vi "Open Reference (Simulate).vi"(8 "error in (no error)":errorcluster, 11 "Instrument Refnum in":refnum<visa-resource-name>) -> (0 "error out":errorcluster, 3 "Instrument Refnum out":refnum<visa-resource-name>)   [LabVIEW 2012]
doc: "Simulates initializing a hardware reference"
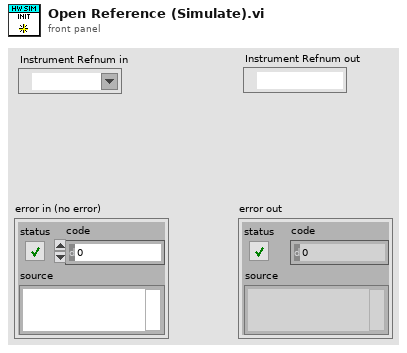
[diagram p1: front panel]
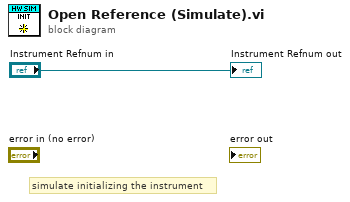
[diagram p0: block diagram]
diagram:
  # "simulate initializing the instrument"
  "Instrument Refnum out" <- "Instrument Refnum in"
